vi "Version Maker.vi"(7 "Version Sheet Cluster":T2={"Folder Path containing version information"=path "", "File name (including .ini)"=path "", "Section"="Simulator"} caption="This is used for automatic verion record.", 8 "Error In":errorcluster, 9 "Open Application Reference in":refnum<vi>, 11 "VI Information":T1) -> (0 "Error Out":errorcluster, 1 "Open Application Reference out":refnum<vi>, 2 "App Name":string, 3 "Standard Config Path":path)   [LabVIEW 2014]
doc: "It is part of HIL Change Management System. \n\nThis VI sets the front panel title, keeps track of the versions of the executable, and registers the executable version in a file that can be used for updating the change registry.\n\nLevel of Application: It is determined as follows: determine the folders for storing .exe and .vi files; find the common parent root and call it level 0. The level of application is determined by the number of levels that you need to go down to see the main VI. \n\nSee the help."
uses:
  <vilib>/Utility/config.llb/Read Key (Boolean).vi
  <vilib>/Utility/config.llb/Write Key (String).vi
  <vilib>/Utility/config.llb/Write Key (Boolean).vi
  <vilib>/Utility/config.llb/Read Key (String).vi
  <vilib>/Utility/config.llb/NI_LVConfig.lvlib
  <vilib>/Utility/file.llb/Write To Spreadsheet File (string).vi
panel:
  # "Change Management System - Version Control"
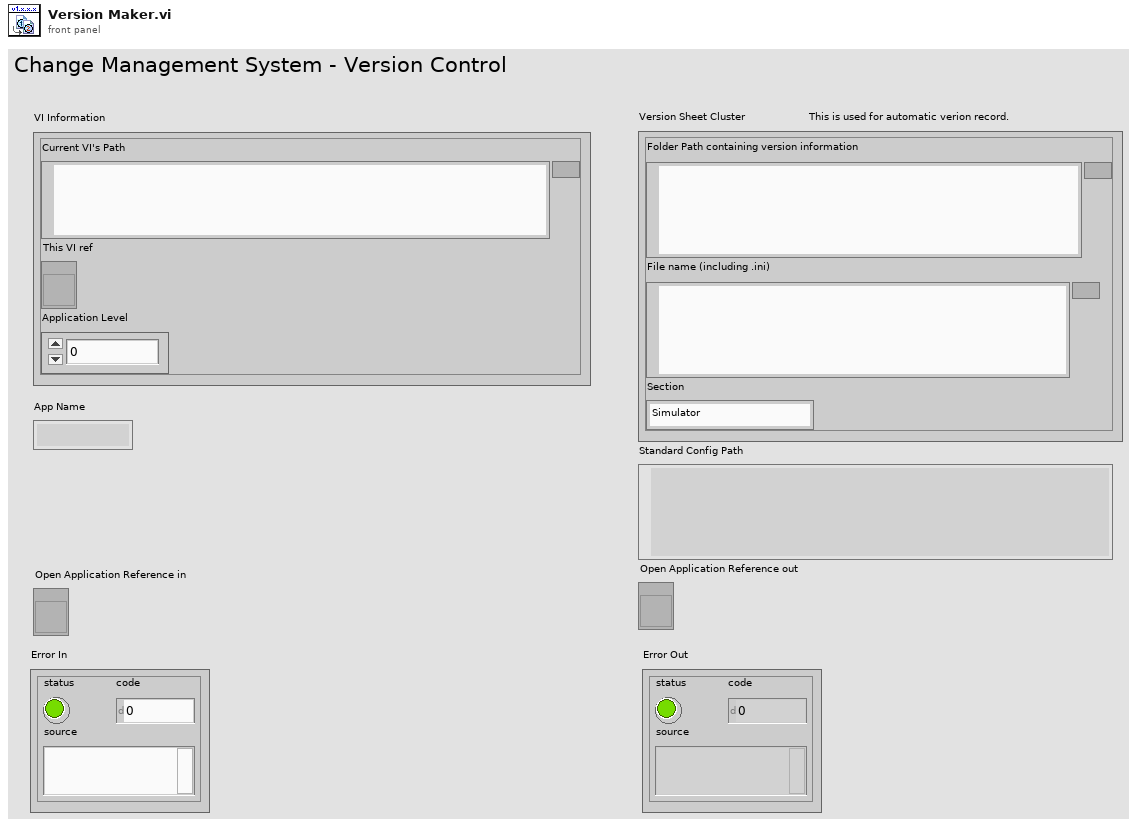
[diagram p1: front panel]
types:
  T1 = cluster{"Current VI's Path":path, "This VI ref":refnum<vi>, "Application Level":u8}
  T2 = cluster{"Folder Path containing version information":path, "File name (including .ini)":path, "Section":string}
  T3 = typedef "NI_LVConfig.lvlib/Config Data RefNum.ctl" = refnum<k1>
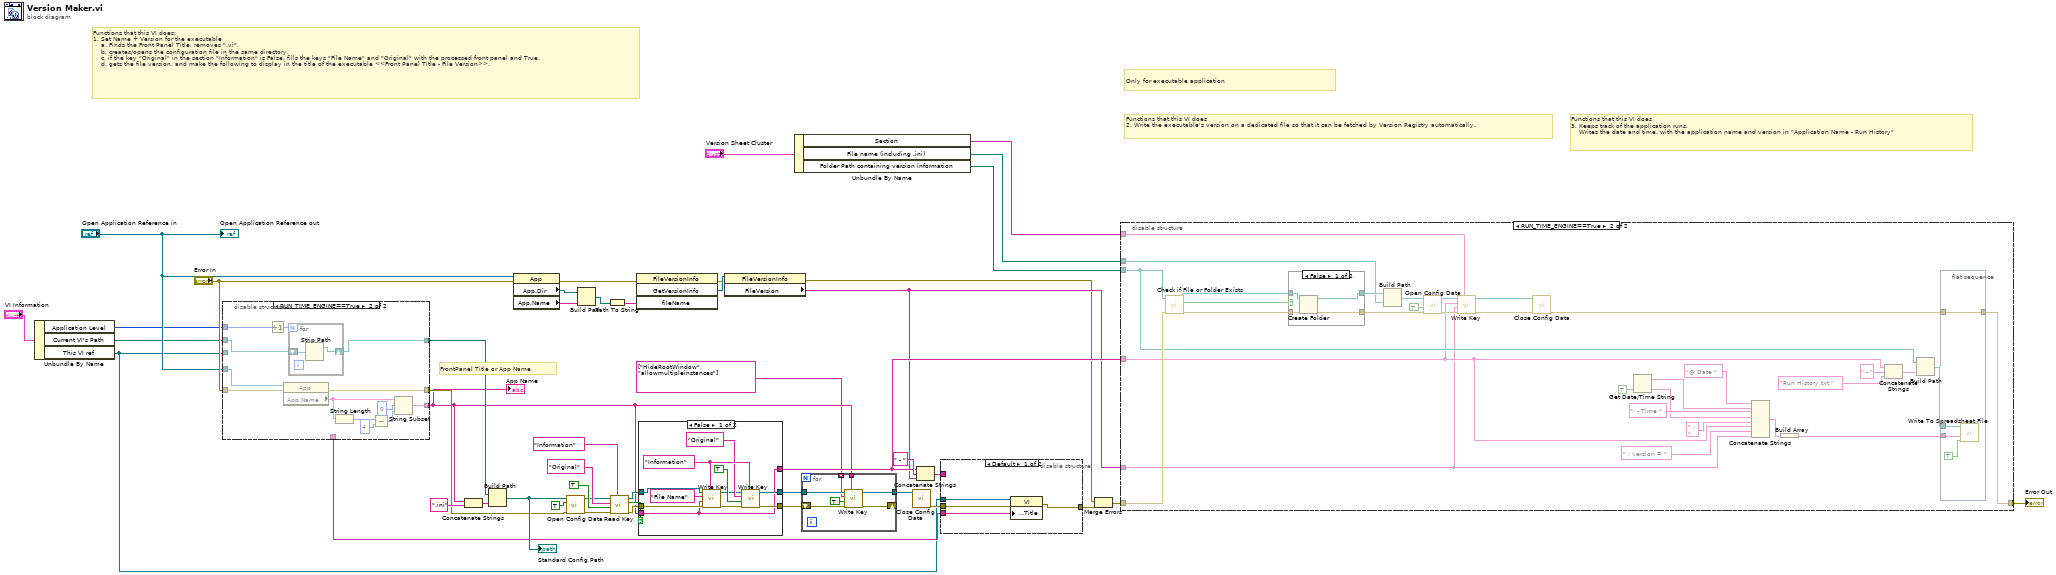
[diagram p0: block diagram]
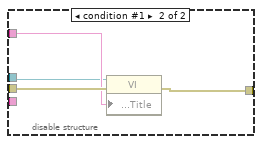
[diagram p4: hidden frame]
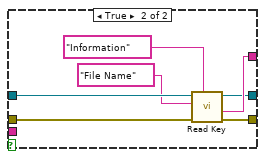
[diagram p5: hidden frame]
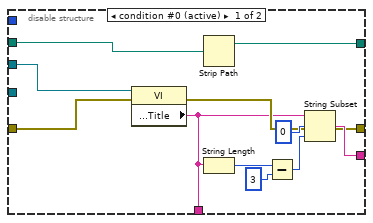
[diagram p6: hidden frame]
diagram:
  # "Only for executable application"
  # "Functions that this VI does\n3. Keeps track of the application runs. \n    Writes the date and time, with the application name and version in \"Application Name - Run History\""
  # "Functions that this VI does\n2. Write the executable's version on a dedicated file so that it can be fetched by Version Registry automatically."
  # "FrontPanel Title or App Name"
  # "Functions that this VI does:\n1. Set Name + Version for the executable\n    a. Finds the Front Panel Title, removes \".vi\", \n    b. creates/opens the configuration file in the same directory, \n    c. if the key \"Original\" in the section \"Information\" is False, fills the keys \"File Name\" and \"Original\" with the processed front panel and True. \n    d. gets the file version, and make the following to display in the title of the executable <<Front Panel Title - File Version>>."
  n1 = Unbundle By Name("VI Information") -> ("Application Level"=w8:u8, "Current VI's Path"=w7:path, "This VI ref"=w6:refnum<vi>)
  n2 = disable-structure shown="RUN_TIME_ENGINE==True" {
    disable-tunnel: w7 -> [w49 w59]
    disable-tunnel: [w57 w58] -> w45
    disable-tunnel: [w52 w65] -> w3
    disable-tunnel: "Error In" -> [w48 w63]
    disable-tunnel: "Open Application Reference in" -> [_ w64]
    disable-tunnel: [w51 w62] -> w22
    disable-tunnel: [w50 _] -> w21
    disable-tunnel: w8 -> [_ w60]
    disable-tunnel: w6 -> [w47 _]
    frame condition #0 (active) {
      n3 = property class="VI"(reference=w47, error in=w48) -> (error out=w51:errorcluster, "Front Panel.Title"=w50:string)  [unwired: 1 out]
      n4 = Strip Path(path=w49) -> (stripped path=w57:path)  [unwired: 1 out]
      n5 = String Length(string=w50) -> (length=w54:i32)
      n6 = Subtract(x=w54, y=3) -> (x-y=w56:i32)
      n7 = String Subset(string=w50, offset (0)=0, length (rest)=w56) -> (substring=w52:string)
    }
    frame condition #1 {
      n8 = Increment(x=w60) -> (x+1=w61:u8)
      n9 = property class="App"(reference=w64, error in=w63) -> (error out=w62:errorcluster, "App.Name"=w66:string)  [unwired: 1 out]
      n10 = for {
        N: w61 -> [_]
        shift-right: [w72] -> w58
        shift-left: w59 -> [w71]
        n11 = Strip Path(path=w71) -> (stripped path=w72:path)  [unwired: 1 out]
      }
      n12 = String Length(string=w66) -> (length=w68:i32)
      n13 = Subtract(x=w68, y=4) -> (x-y=w70:i32)
      n14 = String Subset(string=w66, offset (0)=0, length (rest)=w70) -> (substring=w65:string)
    }
  }
  "App Name" <- w3
  n15 = Concatenate Strings(w3, ".ini" ("string")) -> (w31:string)
  n16 = Build Path(base path=w45, name or relative path=w31) -> (appended path=w44:path)
  "Standard Config Path" <- w44
  n17 = property class="App"(reference="Open Application Reference in", error in="Error In") -> (error out=w27:errorcluster, "App.Dir"=w16:path, "App.Name"=w15:string)  [unwired: 1 out]
  n18 = call <vilib>:"Open Config Data.vi"("error in (no error)"=w22, "create file if necessary (T)"=TRUE, "configuration file path"=w44) -> ("error out"=w28:errorcluster, "refnum"=w29:T3)  [unwired: 6 in, 1 out]
  n19 = Build Path(base path=w16, name or relative path=w15) -> (appended path=w34:path)
  n20 = Path To String(path=w34) -> (string=w33:string)
  n21 = call-poly <vilib>:"Read Key.vi"("section"="Information", "error in (no error)"=w28, "default value"=TRUE ("create file if necessary (T)"), "key"="Original", "refnum"=w29) -> ("error out"=w39:errorcluster, "found?"=w40:bool, "refnum out"=w38:T3)  [unwired: 3 in, 1 out]
  n22 = invoke class="FileVersionInfo" method="GetVersionInfo"(error in=w27, "fileName"=w33) -> (error out=w26:errorcluster, "GetVersionInfo"=w35:refnum<k24>)  [unwired: 2 in, 2 out]
  n23 = case shown="False" w40 {
    tunnel: w39 -> [w83 w89]
    tunnel: w38 -> [w82 w90]
    tunnel: [w75 w87] -> w5
    tunnel: [w74 w86] -> w4
    tunnel: w3 -> [w73 _]
    tunnel: [w73 w88] -> w25
    frame False {
      w80 = "Information" ("section")
      n24 = call-poly <vilib>:"Write Key.vi"("section"=w80, "error in (no error)"=w83, "value"=w73, "key"="File Name", "refnum"=w82) -> ("error out"=w77:errorcluster, "refnum out"=w76:T3)  [unwired: 4 in, 1 out]
      n25 = call-poly <vilib>:"Write Key.vi"("section"=w80, "error in (no error)"=w77, "value"=TRUE ("create file if necessary (T)"), "key"="Original", "refnum"=w76) -> ("error out"=w74:errorcluster, "refnum out"=w75:T3)  [unwired: 4 in, 1 out]
    }
    frame True {
      n26 = call-poly <vilib>:"Read Key.vi"("section"="Information", "error in (no error)"=w89, "key"="File Name", "refnum"=w90) -> ("error out"=w86:errorcluster, "value"=w88:string, "refnum out"=w87:T3)  [unwired: 4 in, 1 out]
    }
  }
  n27 = property class="FileVersionInfo"(reference=w35, error in=w26) -> (error out=w19:errorcluster, "FileVersion"=w24:string)  [unwired: 1 out]
  n28 = Unbundle By Name("Version Sheet Cluster") -> ("Section"=w13:string, "File name (including .ini)"=w11:path, "Folder Path containing version information"=w12:path)
  n29 = for {
    tunnel: w5 -> [w94]
    shift-right: [w96] -> _
    shift-left: w4 -> [w97]
    tunnel: w3 -> [w95]
    tunnel: [w93] -> w2
    tunnel: string[] ["HideRootWindow", "allowmultipleinstances"] -> [w91] mode=indexing
    n30 = call-poly <vilib>:"Write Key.vi"("section"=w95, "error in (no error)"=w97, "value"=TRUE, "key"=w91, "refnum"=w94) -> ("error out"=w96:errorcluster, "refnum out"=w93:T3)  [unwired: 4 in, 1 out]
  }
  n31 = call <vilib>:"Close Config Data.vi"("refnum"=w2) -> ("error out"=w37:errorcluster)  [unwired: 9 in, 1 out]
  n32 = Concatenate Strings(w25, " - " ("section"), w24) -> (w32:string)
  n33 = disable-structure shown="Default" {
    disable-tunnel: w37 -> [w101 w105]
    disable-tunnel: w32 -> [_ w104]
    disable-tunnel: [w99 w103] -> w20
    disable-tunnel: w21 -> [w100 _]
    disable-tunnel: w6 -> [w98 w102]
    frame condition #0 (active) {
      n34 = property class="VI"(reference=w98, error in=w101, "Front Panel.Title"=w100) -> (error out=w99:errorcluster)  [unwired: 1 out]
    }
    frame condition #1 {
      n35 = property class="VI"(reference=w102, error in=w105, "Front Panel.Title"=w104) -> (error out=w103:errorcluster)  [unwired: 1 out]
    }
  }
  n36 = Merge Errors(w19, w20) -> (w18:errorcluster)
  n37 = disable-structure shown="RUN_TIME_ENGINE==True" {
    disable-tunnel: w25 -> [_ w108]
    disable-tunnel: w24 -> [_ w107]
    disable-tunnel: w18 -> [w106 w113]
    disable-tunnel: w11 -> [_ w114]
    disable-tunnel: w12 -> [_ w112]
    disable-tunnel: [w106 w110] -> w17
    disable-tunnel: w13 -> [_ w109]
    frame condition #0 (active) {
    }
    frame condition #1 {
      n38 = call <vilib>:"Check if File or Folder Exists.vi"("error in (no error)"=w113, "path"=w112) -> ("error out"=w122:errorcluster, "file or folder exists?"=w123:bool, "dup path"=w124:path)  [unwired: 7 in]
      n39 = case shown="False" w123 {
        tunnel: [w142 w144] -> w116
        tunnel: w124 -> [w141 w144]
        tunnel: w122 -> [w140 w143]
        tunnel: [w139 w143] -> w115
        frame False {
          n40 = Create Folder(path (use dialog)=w141, error in=w140) -> (created path=w142:path, error out=w139:errorcluster)  [unwired: 1 in, 1 out]
        }
        frame True {
        }
      }
      n41 = Build Path(base path=w116, name or relative path=w114) -> (appended path=w120:path)
      n42 = call <vilib>:"Open Config Data.vi"("error in (no error)"=w115, "create file if necessary (T)"=TRUE, "configuration file path"=w120) -> ("error out"=w125:errorcluster, "refnum"=w119:T3)  [unwired: 6 in, 1 out]
      n43 = call-poly <vilib>:"Write Key.vi"("section"=w109, "error in (no error)"=w125, "value"=w107, "key"=w108, "refnum"=w119) -> ("error out"=w117:errorcluster, "refnum out"=w118:T3)  [unwired: 4 in, 1 out]
      n44 = call <vilib>:"Close Config Data.vi"("error in (no error)"=w117, "refnum"=w118) -> ("error out"=w111:errorcluster)  [unwired: 8 in, 1 out]
      n45 = Get Date/Time String(want seconds? (F)=TRUE) -> (date string=w130:string, time string=w128:string)  [unwired: 2 in]
      n46 = Concatenate Strings("@ Date " ("section"), w130, "  - Time " ("section"), w128, " ; " ("section"), w108, " ; version = " ("section"), w107) -> (w134:string)
      n47 = Build Array(w134) -> (w133:string[])
      n48 = Concatenate Strings(w108, " - " ("section"), "Run History.txt " ("section")) -> (w138:string)
      n49 = Build Path(base path=w112, name or relative path=w138) -> (appended path=w135:path)
      n50 = flat-sequence {
        tunnel: w135 -> [w148]
        tunnel: w133 -> [w146]
        tunnel: [w145] -> w110
        tunnel: w111 -> [w145]
        frame #0 {
          n51 = call-poly <vilib>:"Write To Spreadsheet File.vi"("append to file? (new file:F)"=TRUE, "1D data"=w146, "file path (dialog if empty)"=w148) -> ()  [unwired: 5 in, 1 out]
        }
      }
    }
  }
  "Error Out" <- w17
  "Open Application Reference out" <- "Open Application Reference in"
